vi "gxml_GetEnumTxt.vi"(8 "error in":errorcluster, 10 "Enum":variant) -> (0 "error out":errorcluster, 1 "String Value":string, 2 "SelectionNum":string)   [LabVIEW 2011, in "Third Party VIs.lvlib" / "GXML.lvlib"]
uses:
  GXML.lvlib
  <vilib>/Utility/VariantDataType/VariantType.lvlib
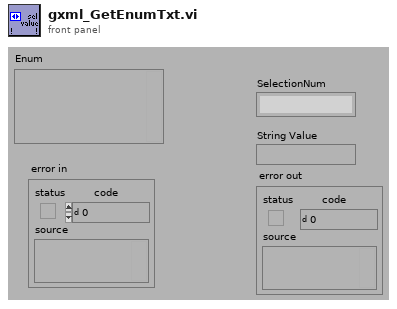
[diagram p1: front panel]
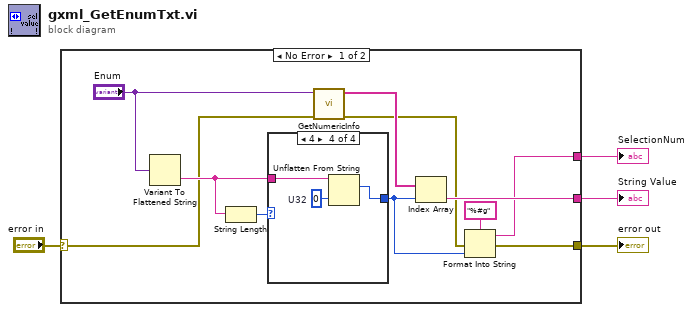
[diagram p0: block diagram]
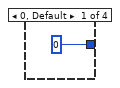
[diagram p2: hidden frame]
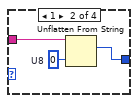
[diagram p3: hidden frame]
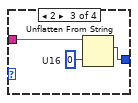
[diagram p4: hidden frame]
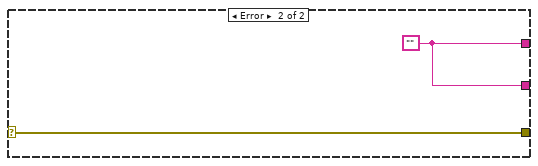
[diagram p5: hidden frame]
diagram:
  n1 = case shown="No Error" "error in" {
    selector: "error in" -> [w5 w27]
    tunnel: [w15 w27] -> w4
    tunnel: [w14 w26] -> w2
    tunnel: [w12 w26] -> w1
    frame No Error {
      n2 = Variant To Flattened String(Variant="Enum") -> (data string=w13:string)  [unwired: 1 out]
      n3 = String Length(string=w13) -> (length=w10:i32)
      n4 = case shown="4" w10 {
        tunnel: w13 -> [_ w19 w22 w25]
        tunnel: [u32 0 ("U32") w17 w20 w23] -> w8
        frame 0, Default {
        }
        frame 1 {
          w18 = u8 0  # U8
          n5 = Unflatten From String(type=w18, binary string=w19) -> (value=w17:u8)  [unwired: 3 in, 2 out]
        }
        frame 2 {
          w21 = u16 0  # U16
          n6 = Unflatten From String(type=w21, binary string=w22) -> (value=w20:u16)  [unwired: 3 in, 2 out]
        }
        frame 4 {
          w24 = u32 0  # U32
          n7 = Unflatten From String(type=w24, binary string=w25) -> (value=w23:u32)  [unwired: 3 in, 2 out]
        }
      }
      n8 = call <vilib>:"GetNumericInfo.vi"("error in (no error)"=w5, "Variant"="Enum") -> ("error out"=w6:errorcluster, "EnumNames"=w7:string[])  [unwired: 6 in, 2 out]
      n9 = Index Array(array=w7, index=w8) -> (element=w14:string)
      n10 = Format Into String(format string="%#g", error in=w6, w8) -> (resulting string=w12:string, error out=w15:errorcluster)  [unwired: 1 in]
    }
    frame Error {
      w26 = ""
    }
  }
  "error out" <- w4
  "String Value" <- w2
  "SelectionNum" <- w1
